vi "CheckShutDown.vi"(11 "statemachine in":refnum<class "statemachine.lvclass">) -> (2 "shutdown":bool)   [LabVIEW 2020, in "eos.lvlib" / "statemachine.lvclass"]
uses:
  statemachine.lvclass
  states/shutting-down/shuttingDown.lvclass
  statemachine.lvclass/statemachine.ctl
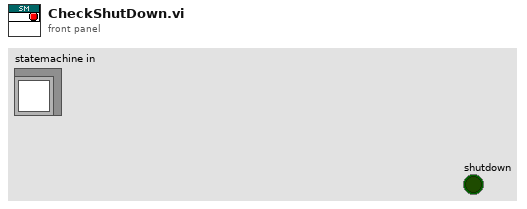
[diagram p1: front panel]
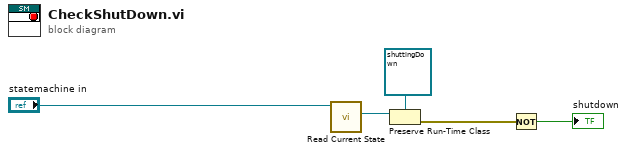
[diagram p0: block diagram]
diagram:
  n1 = call "Read Current State.vi"("statemachine in"="statemachine in") -> ("Current State"=w2:refnum<class "state.lvclass">)  [unwired: 9 in, 1 out]
  n2 = Preserve Run-Time Class(object in=w2, 2:refnum<class "shuttingDown.lvclass"> refnum ("eos.lvlib:shuttingDown.lvclass")) -> (error out=w3:errorcluster)  [unwired: 1 in, 1 out]
  n3 = Not(x=w3) -> (.not. x?=→"shutdown":bool)
